vi "Blend Colors.vi"(9 "blend ratio":dbl=0.5 step=0.01, 10 "onColor":u32(colorbox), 11 "Color":u32(colorbox)) -> (2 "Modified Color":u32(colorbox))   [LabVIEW 2021, in "TSC Material Theme.lvlib" / "Material-Scheme.lvclass"]
doc: "blend the colors together with a blend ratio\n\n<b>Code Developed By:</b>\nTechnology Service Corporation\nwww.tsc.com/atcs\n\nDeveloper:\nDaniel Coons"
uses:
  Material-Scheme.lvclass
panel:
  out "b":u8
  out "g":u8
  out "r":u8
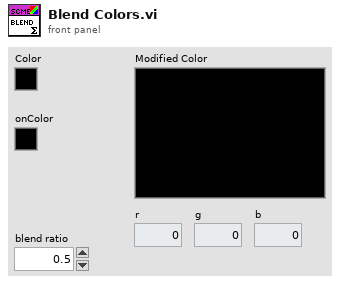
[diagram p1: front panel]
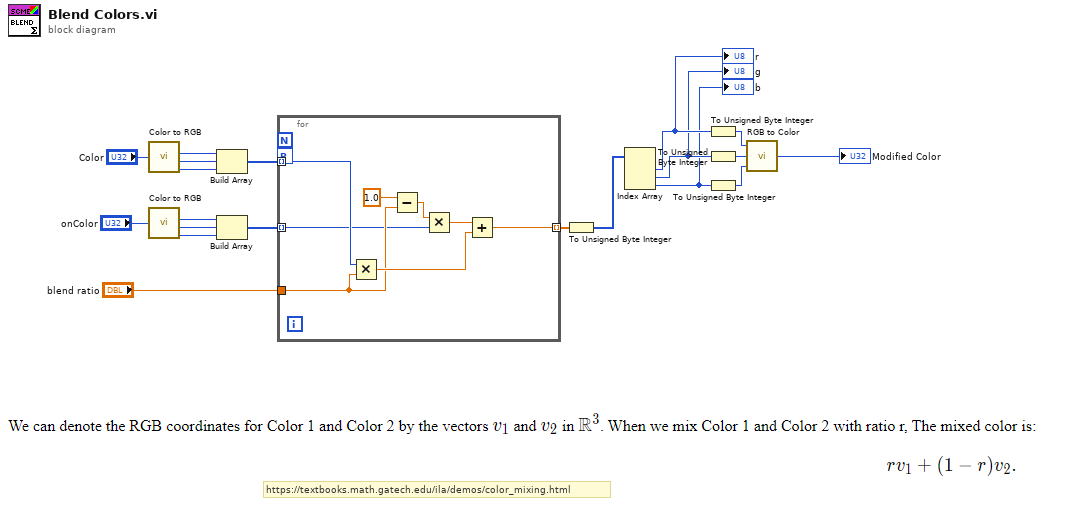
[diagram p0: block diagram]
diagram:
  # "https://textbooks.math.gatech.edu/ila/demos/color_mixing.html"
  n1 = call <vilib>:"Color to RGB.vi"("Color"="Color") -> ("R"=w14:u8, "G"=w8:u8, "B"=w7:u8)  [unwired: 1 out]
  n2 = call <vilib>:"Color to RGB.vi"("Color"="onColor") -> ("R"=w5:u8, "G"=w4:u8, "B"=w3:u8)  [unwired: 1 out]
  n3 = Build Array(w14, w8, w7) -> (w9:u8[])
  n4 = Build Array(w5, w4, w3) -> (w6:u8[])
  n5 = for {
    tunnel: w9 -> [w26] mode=indexing
    tunnel: w6 -> [w21] mode=indexing
    tunnel: "blend ratio" -> [w22]
    tunnel: [w23] -> w13 mode=indexing
    workers-P: _ -> [_]
    n6 = Multiply(x=w26, y=w22) -> (x*y=w28:dbl)
    n7 = Subtract(x=1.0, y=w22) -> (x-y=w24:dbl)
    n8 = Multiply(x=w24, y=w21) -> (x*y=w25:dbl)
    n9 = Add(x=w25, y=w28) -> (x+y=w23:dbl)
  }
  n10 = To Unsigned Byte Integer(number=w13) -> (unsigned 8bit integer=w11:u8[])
  n11 = Index Array(array=w11) -> (element #1=w10:u8, element #2=w2:u8, element #3=w1:u8)  [unwired: 3 in]
  "r" <- w10
  "g" <- w2
  "b" <- w1
  n12 = To Unsigned Byte Integer(number=w10) -> (unsigned 8bit integer=w16:u8)
  n13 = To Unsigned Byte Integer(number=w2) -> (unsigned 8bit integer=w18:u8)
  n14 = To Unsigned Byte Integer(number=w1) -> (unsigned 8bit integer=w19:u8)
  n15 = call <vilib>:"RGB to Color.vi"("B"=w19, "G"=w18, "R"=w16) -> ("Color"=→"Modified Color":u32)
